vi "Security System.vi"() -> ()   [LabVIEW 2013]
doc: "This VI simulates the security system by monitoring the alarm switches, bypass switches, tamper switches and indicates the corresponding activity with different colours."
uses:
  Controls/Security System Indicators.ctl
  Controls/Security System States.ctl
  Controls/Security log States.ctl
  Controls/Security Zones.ctl
panel:
  in  "stop":bool
  out "Zone status indicators":T1
  in  "Tamper switches":bool[](array[boolean])
  in  "Bypass Switches":bool[](array[boolean])
  in  "Alarm Switches":bool[](array[boolean])
  # "· Green: Normal\n· Red: Alarm\n· Blue: Bypass\n· Orange: Tampe"
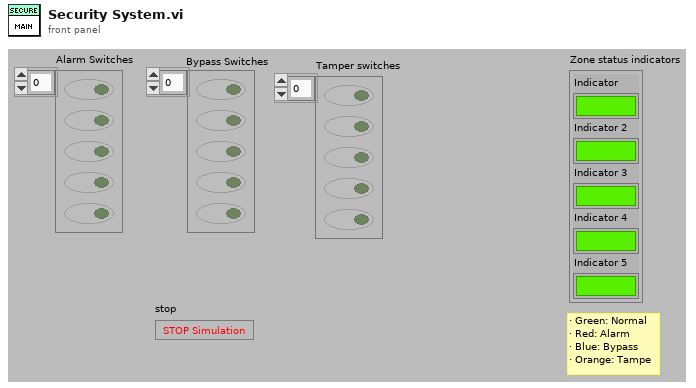
[diagram p1: front panel]
types:
  T1 = typedef "Security System Indicators.ctl" = cluster{"Indicator":bool, "Indicator 2":bool, "Indicator 3":bool, "Indicator 4":bool, "Indicator 5":bool}
  T2 = typedef "Security System States.ctl" = enum16{"Initialize", "Main", "Stop"}
  T3 = typedef "Security log States.ctl" = enum16{"Initialize", "Write", "Close"}
  T4 = typedef "Security Zones.ctl" = enum16{"Normal", "Alarm", "Bypass", "Tamper"}
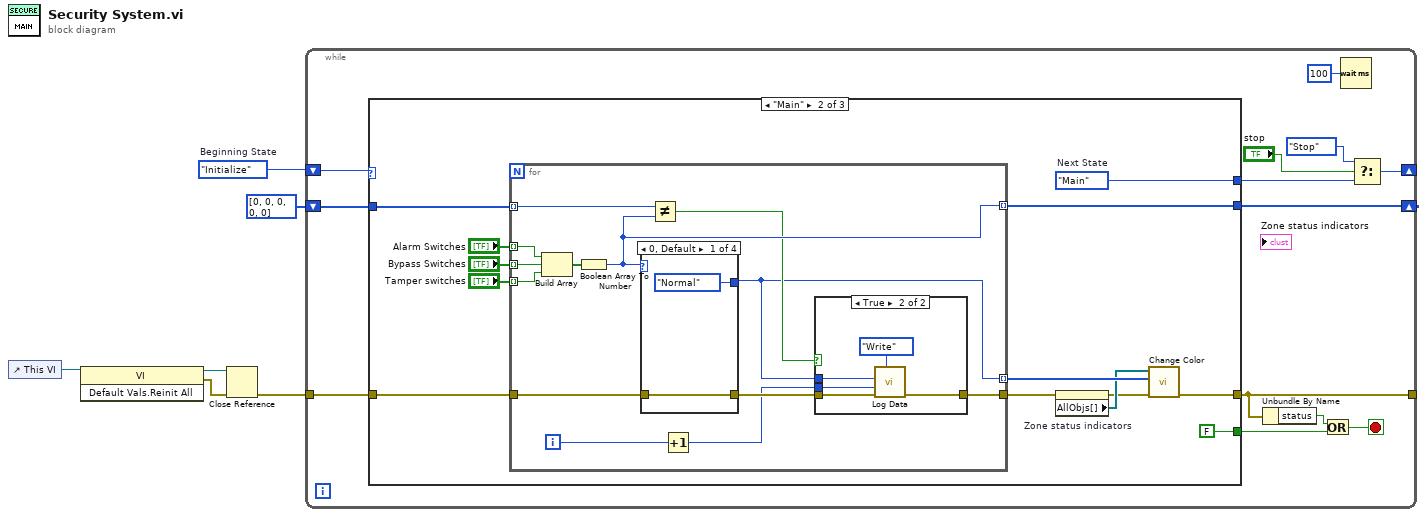
[diagram p0: block diagram]
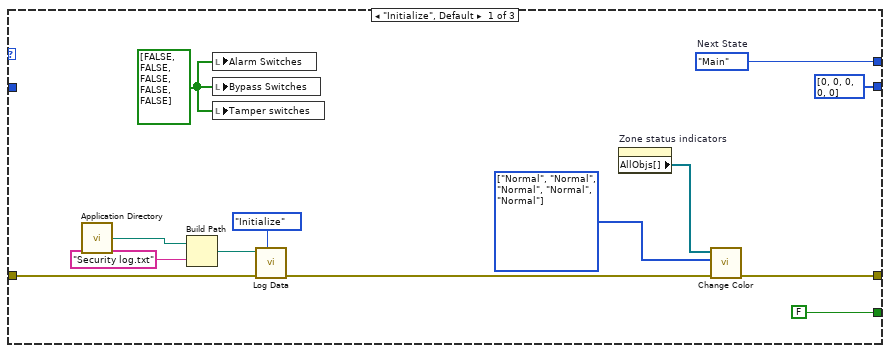
[diagram p2: hidden frame]
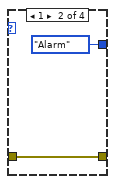
[diagram p4: hidden frame]
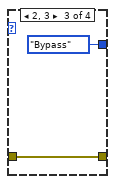
[diagram p5: hidden frame]
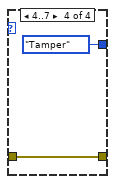
[diagram p6: hidden frame]
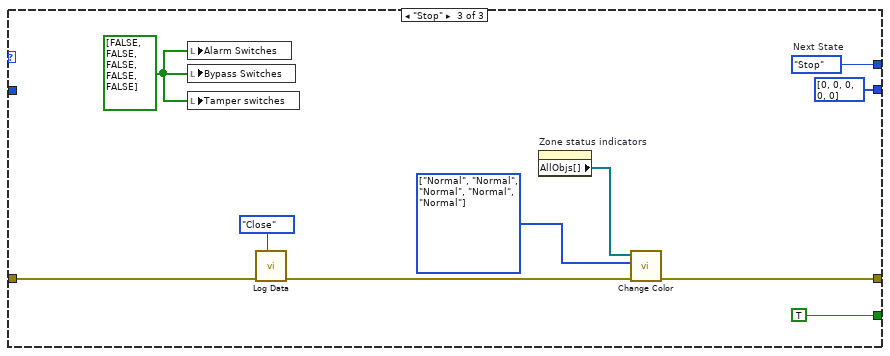
[diagram p7: hidden frame]
diagram:
  w6 = Security_System_States."Initialize"  # Beginning State
  n1 = control-ref of="This VI"() -> (w5:refnum<vi>)
  n2 = invoke class="VI" method="Default Vals.Reinit All"(reference=w5) -> (reference out=w4:refnum<vi>, error out=w3:errorcluster)  [unwired: 2 in, 1 out]
  n3 = Close Reference(reference=w4, error in (no error)=w3) -> (error out=w2:errorcluster)
  n4 = while {
    shift-right: [w11] -> _
    shift-left: w6 -> [w19]
    tunnel: w2 -> [w16]
    tunnel: [w15] -> _
    shift-right: [w8] -> _
    shift-left: u32[] [0, 0, 0, 0, 0] -> [w7]
    stop <- w12 stop-if-true
    n5 = case shown="\"Main\"" w19 {
      tunnel: [w32 w45 w82] -> w18
      tunnel: w16 -> [w30 w40 w80]
      tunnel: [w24 w38 w77] -> w15
      tunnel: [FALSE FALSE TRUE] -> w13
      tunnel: [u32[] [0, 0, 0, 0, 0] w34 u32[] [0, 0, 0, 0, 0]] -> w8
      tunnel: w7 -> [_ w33 _]
      frame "Initialize", Default {
        w21 = T4[] [enum."Normal", enum."Normal", enum."Normal", enum."Normal", enum."Normal"] items=["Normal", "Alarm", "Bypass", "Tamper"]
        w22 = bool[] [FALSE, FALSE, FALSE, FALSE, FALSE] ("Alarm Switches")
        w32 = Security_System_States."Main"  # Next State
        n6 = call <vilib>:"Application Directory.vi"() -> ("Application Directory"=w28:path)
        n7 = Build Path(base path=w28, name or relative path="Security log.txt" ("text")) -> (appended path=w26:path)
        n8 = local write "Alarm Switches"(w22) -> ()
        n9 = local write "Bypass Switches"(w22) -> ()
        n10 = local write "Tamper switches"(w22) -> ()
        n11 = call "Log Data.vi"("Command"=Security_log_States."Initialize", "error in (no error)"=w30, "file path"=w26) -> ("error out"=w25:errorcluster)  [unwired: 8 in]
        n12 = property on="Zone status indicators" class="Clust (strict)"() -> ("AllObjs[]"=w23:refnum<vi>[])  [unwired: 2 in, 2 out]
        n13 = call "Change Color.vi"("error in (no error)"=w25, "Status"=w21, "AllObjs[]"=w23) -> ("error out"=w24:errorcluster)  [unwired: 8 in]
      }
      frame "Main" {
        w45 = Security_System_States."Main"  # Next State
        n14 = for {
          tunnel: "Alarm Switches" -> [w58] mode=indexing
          tunnel: "Bypass Switches" -> [w57] mode=indexing
          tunnel: "Tamper switches" -> [w56] mode=indexing
          tunnel: [w52] -> w36
          tunnel: w40 -> [w54]
          tunnel: [w48] -> w39 mode=indexing
          tunnel: [w50] -> w34 mode=indexing
          tunnel: w33 -> [w51] mode=indexing
          i -> [w47]
          n15 = Build Array(w58, w57, w56) -> (w55:bool[])
          n16 = Boolean Array To Number(Boolean array=w55) -> (number=w50:u32)
          n17 = case shown="0, Default" w50 {
            tunnel: w54 -> [w66 w68 w70 w72]
            tunnel: [w66 w68 w70 w72] -> w53
            tunnel: [Security_Zones."Normal" ("Status") Security_Zones."Alarm" ("Status") Security_Zones."Bypass" ("Status") Security_Zones."Tamper" ("Status")] -> w48
            frame 0, Default {
            }
            frame 1 {
            }
            frame 2, 3 {
            }
            frame 4..7 {
            }
          }
          n18 = Not Equal?(x=w51, y=w50) -> (x != y?=w49:bool)
          n19 = Increment(x=w47) -> (x+1=w46:i32)
          n20 = case shown="True" w49 {
            tunnel: w53 -> [w59 w64]
            tunnel: [w59 w63] -> w52
            tunnel: w48 -> [_ w61]
            tunnel: w46 -> [_ w60]
            frame False {
            }
            frame True {
              n21 = call "Log Data.vi"("Command"=Security_log_States."Write", "error in (no error)"=w64, "Zone"=w60, "Status"=w61) -> ("error out"=w63:errorcluster)  [unwired: 7 in]
            }
          }
        }
        n22 = property on="Zone status indicators" class="Clust (strict)"(error in=w36) -> (error out=w35:errorcluster, "AllObjs[]"=w37:refnum<vi>[])  [unwired: 1 in, 1 out]
        n23 = call "Change Color.vi"("error in (no error)"=w35, "Status"=w39, "AllObjs[]"=w37) -> ("error out"=w38:errorcluster)  [unwired: 8 in]
      }
      frame "Stop" {
        w73 = bool[] [FALSE, FALSE, FALSE, FALSE, FALSE] ("Alarm Switches")
        w75 = T4[] [enum."Normal", enum."Normal", enum."Normal", enum."Normal", enum."Normal"] items=["Normal", "Alarm", "Bypass", "Tamper"]
        w82 = Security_System_States."Stop"  # Next State
        n24 = local write "Alarm Switches"(w73) -> ()
        n25 = local write "Bypass Switches"(w73) -> ()
        n26 = local write "Tamper switches"(w73) -> ()
        n27 = call "Log Data.vi"("Command"=Security_log_States."Close", "error in (no error)"=w80) -> ("error out"=w78:errorcluster)  [unwired: 9 in]
        n28 = property on="Zone status indicators" class="Clust (strict)"() -> ("AllObjs[]"=w76:refnum<vi>[])  [unwired: 2 in, 2 out]
        n29 = call "Change Color.vi"("error in (no error)"=w78, "Status"=w75, "AllObjs[]"=w76) -> ("error out"=w77:errorcluster)  [unwired: 8 in]
      }
    }
    n30 = Unbundle By Name(w15) -> ("status"=w14:bool)
    n31 = Or(x=w14, y=w13) -> (x .or. y?=w12:bool)
    n32 = Wait (ms)(milliseconds to wait=u32 100) -> ()  [unwired: 1 out]
    n33 = Select(t=Security_System_States."Stop" ("Next State"), s="stop", f=w18) -> (s? t:f=w11:T2)
  }
